vi "Array - Failure Message.vi"() -> ()   [LabVIEW 2017, in "Assertions.Tests.lvlib" / "Assert Collection Empty.lvlib"]
uses:
  Assert Collection Empty.lvlib
  cbee6d11-a8dd-48ad-99e8-9ee3396d33d5.vi
  src/Transparent Assertions/Constraints/Collection Is Empty/Collection Is Empty.lvclass
  src/Transparent Assertions/Assertions/Assertions.lvlib
panel:
  out "error out":errorcluster
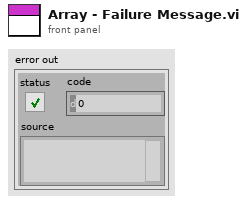
[diagram p1: front panel]
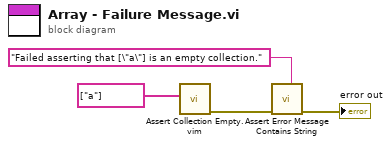
[diagram p0: block diagram]
diagram:
  n1 = call "Assert Collection Empty.vim"("Collection"=string[] ["a"]) -> ("error out"=w3:errorcluster)  [unwired: 10 in]
  n2 = call "Assert Error Message Contains String.vi"("Expected"="Failed asserting that [\"a\"] is an empty collection.", "error in (no error)"=w3) -> ("error out"=→"error out":errorcluster)  [unwired: 9 in]
